vi "S1500_S7Com_Once.vi"() -> ()   [LabVIEW 2018]
doc: "Demonstrates minimalist Reading from or Writing to a PLC, once per execution."
uses:
  S7Com_Source_inkl_IP/S7Com_Data_Array.ctl
  S1500_S7Com_RW_CMD.ctl
  S1500_S7Com_Address_Area.ctl
  S1500_S7Com_Start_Add.ctl
  S1500_S7Com_Transport_Size.ctl
  S1500_S7Com_Function.ctl
panel:
  in  "停止":bool
  out "数值":i32
  in  "RW_CMD":T1={"Read Length"=1, "Data Block #"=1, "S7_Add_Area"=132, "Start Address"=0, "S7_Transport_Size"=2, "S7_Function"=4, "IP-Address"=""} {"S7_Function" items=["Read"=4, "Write"=5]; "S7_Transport_Size" items=["BIT"=1, "BYTE"=2, "CHAR"=3, "WORD"=4, "INT"=5, "DWORD"=6, "DINT"=7, "REAL"=8]; "S7_Add_Area" items=["P Area"=128, "I Area"=129, "O Area"=130, "M Area"=131, "DB Area"=132, "Counter"=40, "Timer"=41]}
  out "Read Data":T6 format="%.0x"
  out "error out":errorcluster
  in  "error in (no error)":errorcluster
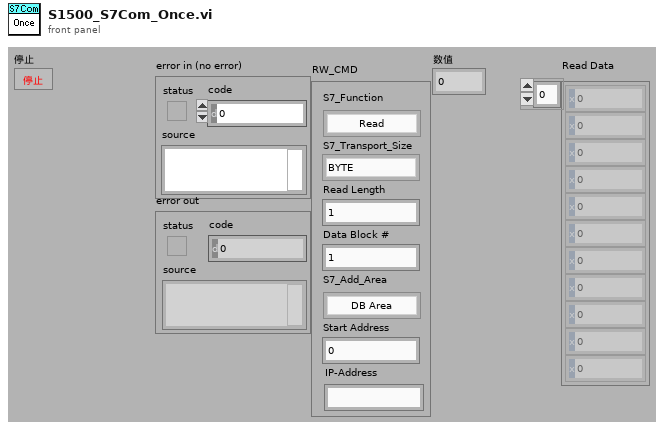
[diagram p1: front panel]
types:
  T1 = typedef "S1500_S7Com_RW_CMD.ctl" = cluster{"Read Length":u16, "Data Block #":u16, "S7_Add_Area":T2, "Start Address":T3, "S7_Transport_Size":T4, "S7_Function":T5, "IP-Address":string}
  T2 = typedef "S1500_S7Com_Address_Area.ctl" = u8
  T3 = typedef "S1500_S7Com_Start_Add.ctl" = u16
  T4 = typedef "S1500_S7Com_Transport_Size.ctl" = u8
  T5 = typedef "S1500_S7Com_Function.ctl" = u8
  T6 = typedef "S7Com_Data_Array.ctl" = i32[]
  T7 = typedef "S1500_S7Com_Data_Array.ctl" = i32[]
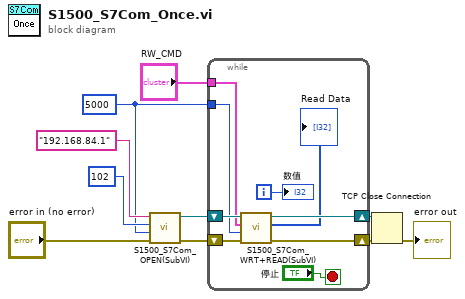
[diagram p0: block diagram]
diagram:
  w2 = 5000 ("timeout ms (5000)")
  n1 = call "S1500_S7Com_OPEN(SubVI).vi"("remote address"="192.168.84.1", "remote port"=u16 102, "timeout ms"=w2, "error in (no error)"="error in (no error)") -> ("connection ID out"=w6:refnum<k5>, "error out"=w3:errorcluster)  [unwired: 3 out]
  n2 = while {
    tunnel: w2 -> [w15]
    tunnel: "RW_CMD" -> [w14]
    shift-right: [w18] -> w5
    shift-left: w6 -> [w19]
    shift-right: [w17] -> w4
    shift-left: w3 -> [w16]
    i -> [w13]
    stop <- "停止" stop-if-true
    n3 = call "S1500_S7Com_WRT+READ(SubVI).vi"("error in"=w16, "timeout ms (25000)"=w15, "RW_CMD"=w14, "connection ID in"=w19) -> ("error out"=w17:errorcluster, "Read_Data"=→"Read Data":T7, "connection ID out"=w18:refnum<k5>)  [unwired: 1 in, 1 out]
    "数值" <- w13
  }
  n4 = TCP Close Connection(connection ID=w5, error in (no error)=w4) -> (error out=→"error out":errorcluster)  [unwired: 2 out]
